vi "ArmGainScheduler.vi"(8 "Lock Setpoint as Current Height":bool, 9 "On Bert?":bool=TRUE, 10 "Have Can?":i8, 11 "Arm States":T2) -> (3 "Arm Gains Out":T1)   [LabVIEW 2014]
uses:
  Typedefs/Arm States.ctl
  Typedefs/StackerStates.ctl
panel:
  in  "Lock Gains":T1={"Arm_kP"=0.5, "Arm_kI"=0.1, "Arm_kD"=0.0, "Cos Theta Kp"=0.0}
  in  "Manual":T1
  in  "Ernie Arm Gain Scheduler Up":T3(array[cluster])=[{"Arm_kP"=0.2, "Arm_kI"=0.1, "Arm_kD"=0.01, "Cos Theta Kp "=0.0}, {"Arm_kP"=0.2, "Arm_kI"=0.1, "Arm_kD"=0.01, "Cos Theta Kp "=0.0}, {"Arm_kP"=0.0, "Arm_kI"=0.0, "Arm_kD"=0.0, "Cos Theta Kp "=0.0}, {"Arm_kP"=0.0, "Arm_kI"=0.0, "Arm_kD"=0.0, "Cos Theta Kp "=0.0}, {"Arm_kP"=0.0, "Arm_kI"=0.0, "Arm_kD"=0.0, "Cos Theta Kp "=0.0}, {"Arm_kP"=0.0, "Arm_kI"=0.0, "Arm_kD"=0.0, "Cos Theta Kp "=0.0}, {"Arm_kP"=0.0, "Arm_kI"=0.0, "Arm_kD"=0.0, "Cos Theta Kp "=0.0}]
  in  "Ernie Arm Gain Scheduler Down":T3(array[cluster])=[{"Arm_kP"=0.2, "Arm_kI"=0.1, "Arm_kD"=0.01, "Cos Theta Kp "=0.0}, {"Arm_kP"=0.2, "Arm_kI"=0.1, "Arm_kD"=0.01, "Cos Theta Kp "=0.0}, {"Arm_kP"=0.0, "Arm_kI"=0.0, "Arm_kD"=0.0, "Cos Theta Kp "=0.0}, {"Arm_kP"=0.0, "Arm_kI"=0.0, "Arm_kD"=0.0, "Cos Theta Kp "=0.0}, {"Arm_kP"=0.0, "Arm_kI"=0.0, "Arm_kD"=0.0, "Cos Theta Kp "=0.0}, {"Arm_kP"=0.0, "Arm_kI"=0.0, "Arm_kD"=0.0, "Cos Theta Kp "=0.0}, {"Arm_kP"=0.0, "Arm_kI"=0.0, "Arm_kD"=0.0, "Cos Theta Kp "=0.0}]
  in  "Travel Direction Up":bool
  in  "Bert Arm Gain Scheduler Up":T3(array[cluster])=[{"Arm_kP"=0.2, "Arm_kI"=0.1, "Arm_kD"=0.01, "Cos Theta Kp "=0.0}, {"Arm_kP"=0.2, "Arm_kI"=0.1, "Arm_kD"=0.01, "Cos Theta Kp "=0.0}, {"Arm_kP"=0.0, "Arm_kI"=0.0, "Arm_kD"=0.0, "Cos Theta Kp "=0.0}, {"Arm_kP"=0.0, "Arm_kI"=0.0, "Arm_kD"=0.0, "Cos Theta Kp "=0.0}, {"Arm_kP"=0.0, "Arm_kI"=0.0, "Arm_kD"=0.0, "Cos Theta Kp "=0.0}, {"Arm_kP"=0.0, "Arm_kI"=0.0, "Arm_kD"=0.0, "Cos Theta Kp "=0.0}, {"Arm_kP"=0.0, "Arm_kI"=0.0, "Arm_kD"=0.0, "Cos Theta Kp "=0.0}]
  in  "Bert Arm Gain Scheduler Down":T3(array[cluster])=[{"Arm_kP"=0.2, "Arm_kI"=0.1, "Arm_kD"=0.01, "Cos Theta Kp "=0.0}, {"Arm_kP"=0.2, "Arm_kI"=0.1, "Arm_kD"=0.01, "Cos Theta Kp "=0.0}, {"Arm_kP"=0.0, "Arm_kI"=0.0, "Arm_kD"=0.0, "Cos Theta Kp "=0.0}, {"Arm_kP"=0.0, "Arm_kI"=0.0, "Arm_kD"=0.0, "Cos Theta Kp "=0.0}, {"Arm_kP"=0.0, "Arm_kI"=0.0, "Arm_kD"=0.0, "Cos Theta Kp "=0.0}, {"Arm_kP"=0.0, "Arm_kI"=0.0, "Arm_kD"=0.0, "Cos Theta Kp "=0.0}, {"Arm_kP"=0.0, "Arm_kI"=0.0, "Arm_kD"=0.0, "Cos Theta Kp "=0.0}]
  # "0 is no can\n\n1 is have can"
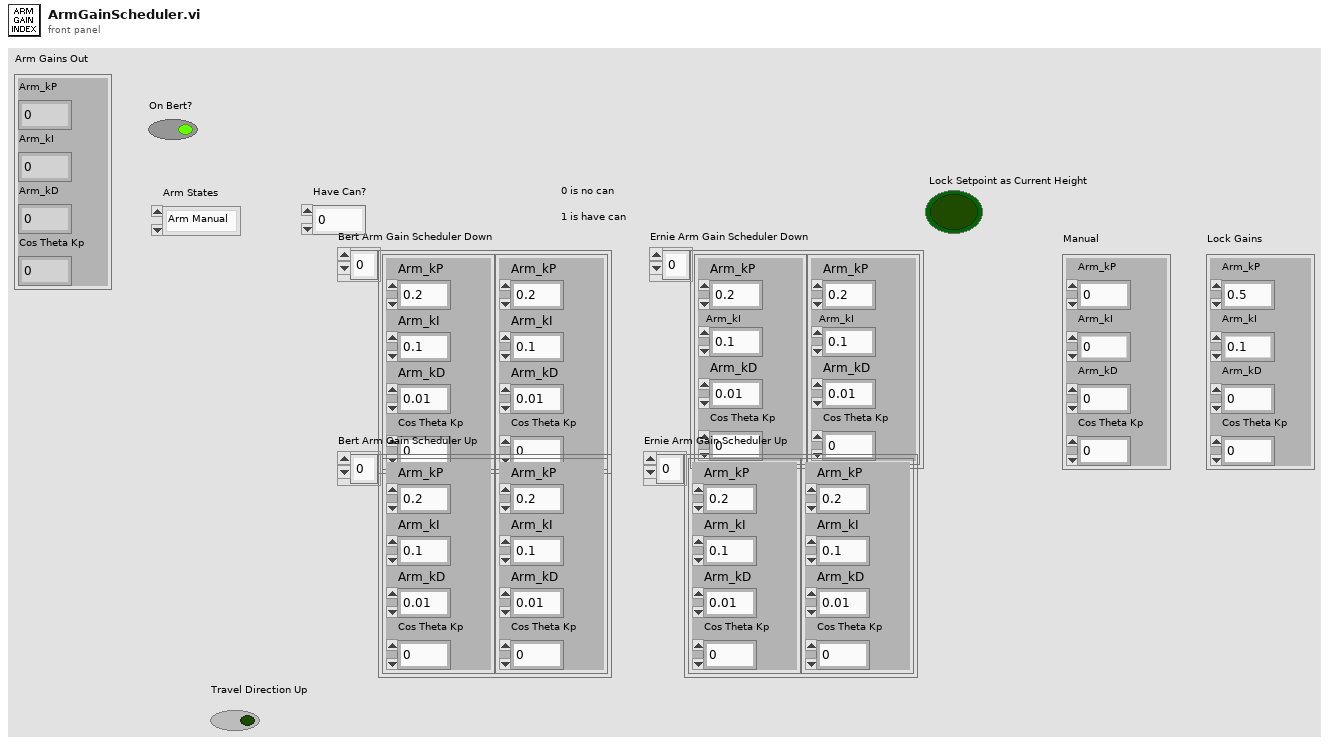
[diagram p1: front panel]
types:
  T1 = cluster{"Arm_kP":dbl, "Arm_kI":dbl, "Arm_kD":dbl, "Cos Theta Kp":dbl}
  T2 = typedef "Arm States.ctl" = enum16{"Arm Manual ", "Ground", "Step", "1 Tote", "2 Tote", "3 Tote", "4 Tote", "5 Tote", "6 Tote", "Flip Can Arm", "Grab Can in auto", "Nudge"}
  T3 = cluster{"Arm_kP":dbl, "Arm_kI":dbl, "Arm_kD":dbl, "Cos Theta Kp ":dbl}[]
  T4 = typedef "StackerStates.ctl" = enum16{"Manual ", "Hold", "Hold5", "Hold6", "GetTote", "DropStack", "Hover", "Hover5", "Wait for Up", "DecideHold", "DownTimerPeriod", "Prep Intake for Drop", "Check Arm before 5", "Make Arm ready for 5", "Check Arm before 6", "Make Arm ready for 6", "Delay for 5", "Delay for 6"}
  T5 = cluster{"Arm_kP":dbl, "Arm_kI":dbl, "Arm_kD":dbl, "Cos Theta Kp ":dbl}
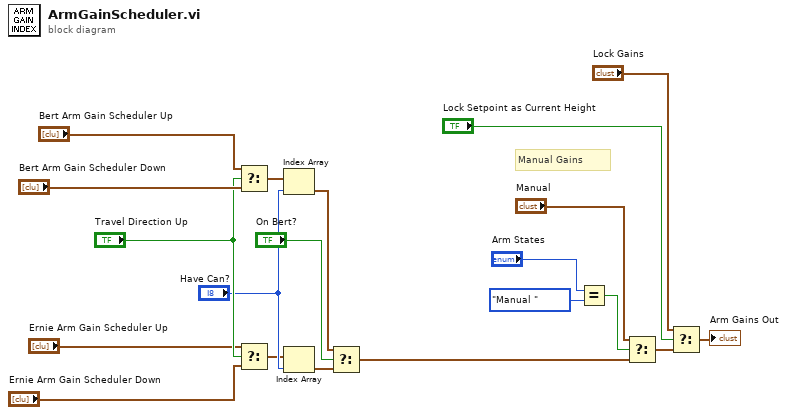
[diagram p0: block diagram]
diagram:
  # "Manual Gains"
  n1 = Select(t="Bert Arm Gain Scheduler Up", s="Travel Direction Up", f="Bert Arm Gain Scheduler Down") -> (s? t:f=w16:T3)
  n2 = Select(t="Ernie Arm Gain Scheduler Up", s="Travel Direction Up", f="Ernie Arm Gain Scheduler Down") -> (s? t:f=w8:T3)
  n3 = Index Array(array=w16, index="Have Can?") -> (element=w15:T5)
  n4 = Index Array(array=w8, index="Have Can?") -> (element=w7:T5)
  n5 = Select(t=w15, s="On Bert?", f=w7) -> (s? t:f=w6:T5)
  n6 = Equal?(x="Arm States", y=StackerStates."Manual " ("StackerState 2")) -> (x = y?=w19:bool)
  n7 = Select(t="Manual", s=w19, f=w6) -> (s? t:f=w4:T5)
  n8 = Select(t="Lock Gains", s="Lock Setpoint as Current Height", f=w4) -> (s? t:f=→"Arm Gains Out":T5)
